vi "solar_app Create Folder.vi"(8 "error in (no error)":errorcluster, 11 "Directory":path) -> (0 "error out":errorcluster, 3 "dup Directory":path)   [LabVIEW 2018]
doc: "This creates a directory if it does not exist."
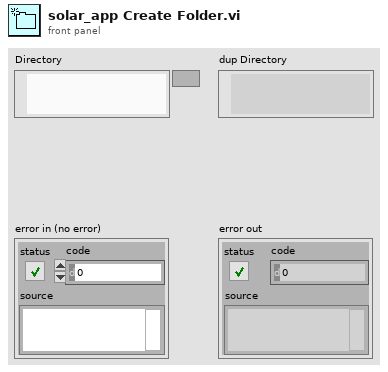
[diagram p1: front panel]
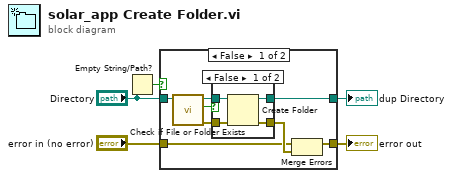
[diagram p0: block diagram]
diagram:
  n1 = Empty String/Path?(string/path="Directory") -> (empty?=w1:bool)
  n2 = case shown="False" w1 {
    tunnel: [w9 w21] -> w5
    tunnel: [w8 w20] -> w4
    tunnel: "error in (no error)" -> [w7 w20]
    tunnel: "Directory" -> [w6 w21]
    frame False {
      n3 = call <vilib>:"Check if File or Folder Exists.vi"("path"=w6) -> ("error out"=w12:errorcluster, "file or folder exists?"=w13:bool, "dup path"=w11:path)  [unwired: 8 in]
      n4 = case shown="False" w13 {
        tunnel: w11 -> [w17 w18]
        tunnel: w12 -> [w16 w19]
        tunnel: [w15 w19] -> w10
        tunnel: [w14 w18] -> w9
        frame False {
          n5 = Create Folder(path (use dialog)=w17, error in=w16) -> (created path=w14:path, error out=w15:errorcluster)  [unwired: 1 in, 1 out]
        }
        frame True {
        }
      }
      n6 = Merge Errors(w7, w10) -> (w8:errorcluster)
    }
    frame True {
    }
  }
  "error out" <- w4
  "dup Directory" <- w5
